vi "RSZVB Start Mixer Delay Calibration Sweep.vi"(8 "error in (no error)":errorcluster {"code" format="%.0x"}, 10 "Channel (1)":i32=1, 11 "VISA session":refnum<visa-resource-name>) -> (0 "error out":errorcluster {"code" format="%.0x"}, 3 "dup VISA session":refnum<visa-resource-name>)   [LabVIEW 2011]
doc: "Starts a calibration sweep for the mixer delay measurement. \n\nNotes:\n\n(1) This mode requires options R&S ZVA-K9 and R&S ZVA-K4\n\nRemote-control command(s):\n[SENSe<Ch>:]FREQuency:MDELay:ACQuire"
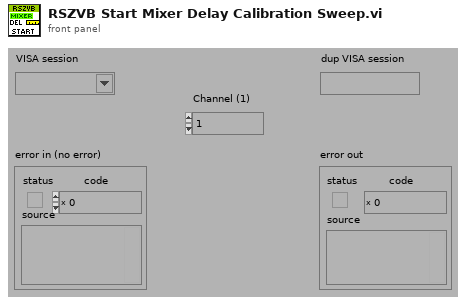
[diagram p1: front panel]
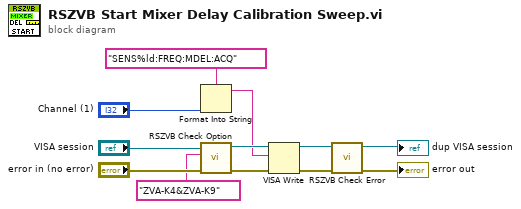
[diagram p0: block diagram]
diagram:
  n1 = Format Into String(format string="SENS%ld:FREQ:MDEL:ACQ", "Channel (1)") -> (resulting string=w5:string)  [unwired: 2 in, 1 out]
  n2 = call "RSZVB Check Option.vi"("error in (no error)"="error in (no error)", "Options"="ZVA-K4&ZVA-K9", "VISA session"="VISA session") -> ("error out"=w7:errorcluster, "dup VISA session"=w6:refnum<visa-resource-name>)  [unwired: 7 in]
  n3 = VISA Write(VISA resource name=w6, write buffer=w5, error in (no error)=w7) -> (VISA resource name out=w3:refnum<visa-resource-name>, error out=w4:errorcluster)  [unwired: 1 out]
  n4 = call "RSZVB Check Error.vi"("error in (no error)"=w4, "VISA session"=w3) -> ("error out"=→"error out":errorcluster, "dup VISA session"=→"dup VISA session":refnum<visa-resource-name>)  [unwired: 8 in]
